vi "Get myRIO PIDs.vi"() -> (3 "myRIO PIDs":u32[](array[numeric]) format="%.0x")   [LabVIEW 2021]
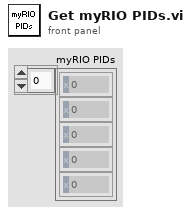
[diagram p1: front panel]
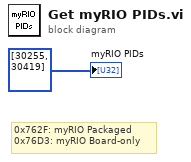
[diagram p0: block diagram]
diagram:
  # "0x762F: myRIO Packaged\n0x76D3: myRIO Board-only"
  "myRIO PIDs" <- u32[] [30255, 30419]
